vi "CheckForMaxNumberOfOpenFiles.vi"(8 "error in (no error)":errorcluster, 9 "data":T1, 10 "data event":T6, 11 "config":T5) -> (0 "error out":errorcluster, 3 "ok to open new file":bool)   [LabVIEW 2017, in "McsaDataEventCreator.lvlib"]
uses:
  <vilib>/addons/InsightCM/Devices/Shared/Mcsa/McsaDataEventCreator/McsaDataEventCreator.lvlib
  <vilib>/addons/InsightCM/Devices/Shared/Mcsa/McsaDataEventCreator/controls/DataEventConfig.ctl
  <vilib>/addons/InsightCM/Devices/Shared/Mcsa/McsaDataEventCreator/controls/AcqParams.ctl
  <vilib>/addons/InsightCM/Devices/Shared/Common/DataAccumulator/controls/AccumulationSettings.ctl
  <vilib>/addons/InsightCM/Devices/Shared/Common/DataAccumulator/controls/accumulationType.ctl
  <vilib>/addons/InsightCM/Devices/Shared/Common/DVRBuffer/controls/BufferLocation.ctl
  <vilib>/addons/PointValueMap/controls/PointMap.ctl
  <vilib>/addons/InsightCM/Devices/Shared/Mcsa/McsaDataEventCreator/controls/config.ctl
  <vilib>/addons/InsightCM/Devices/Shared/Common/DataFlow/controls/Data.ctl
  <vilib>/addons/InsightCM/Utilities/DataAccessors/controls/wfmSGL_DVR.ctl
  <vilib>/addons/InsightCM/Devices/Shared/Common/DataFlow/controls/Type.ctl
  <vilib>/addons/PointValueMap/PointValueMap.lvlib
  <vilib>/addons/InsightCM/Devices/Shared/Common/DVRBuffer/DVRBuffer.lvlib
  <vilib>/addons/InsightCM/Devices/Shared/Common/DataAccumulator/DataAccumulator.lvlib
  <vilib>/addons/InsightCM/Devices/Shared/Common/DataFlow/DataFlow.lvlib
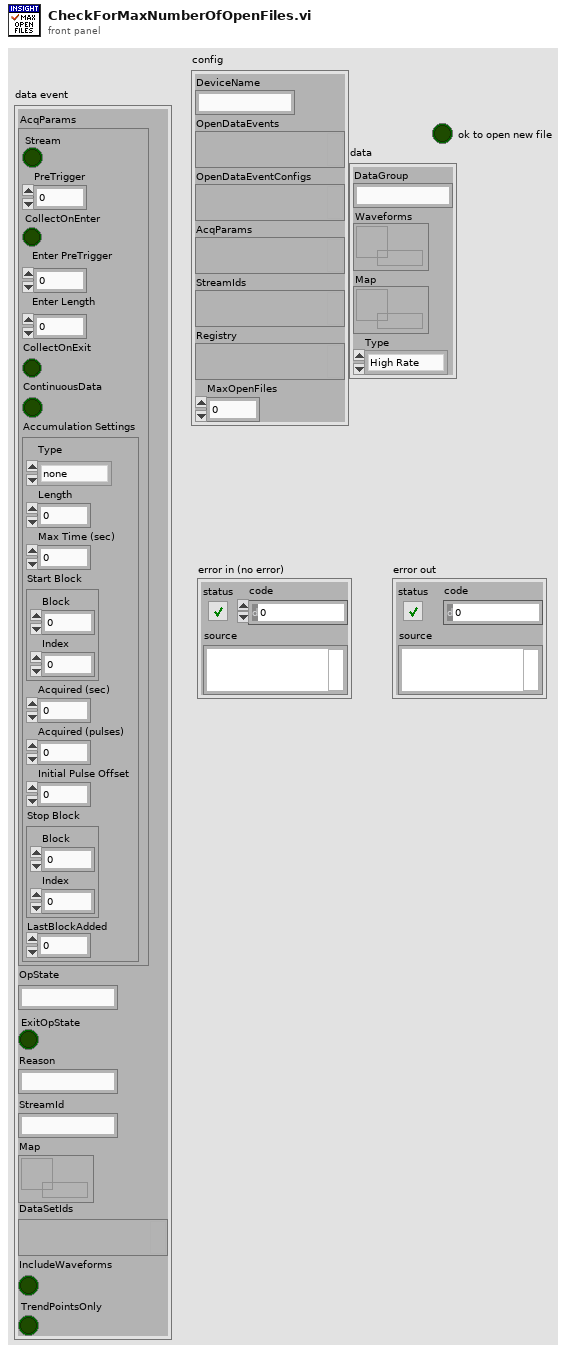
[diagram p1: front panel]
types:
  T1 = typedef "DataFlow.lvlib/Data.ctl" = cluster{"DataGroup":string, "Waveforms":T2, "Map":T3, "Type":T4}
  T2 = typedef "wfmSGL_DVR.ctl" = refnum<data-value>
  T3 = typedef "PointValueMap.lvlib/PointMap.ctl" = refnum<data-value>
  T4 = typedef "DataFlow.lvlib/Type.ctl" = enum16{"High Rate", "Low Rate", "Burst Mode"}
  T5 = typedef "McsaDataEventCreator.lvlib/config.ctl" = cluster{"DeviceName":string, "OpenDataEvents":variant, "OpenDataEventConfigs":variant, "AcqParams":variant, "StreamIds":variant, "Registry":variant, "MaxOpenFiles":i32}
  T6 = typedef "McsaDataEventCreator.lvlib/DataEventConfig.ctl" = cluster{"AcqParams":T7, "OpState":string, "ExitOpState":bool, "Reason":string, "StreamId":string, "Map":T3, "DataSetIds":variant, "IncludeWaveforms":bool, "TrendPointsOnly":bool}
  T7 = typedef "McsaDataEventCreator.lvlib/AcqParams.ctl" = cluster{"Stream":bool, "PreTrigger":i32, "CollectOnEnter":bool, "Enter PreTrigger":i32, "Enter Length":dbl, "CollectOnExit":bool, "ContinuousData":bool, "Accumulation Settings":T8}
  T8 = typedef "DataAccumulator.lvlib/AccumulationSettings.ctl" = cluster{"Type":T9, "Length":dbl, "Max Time (sec)":dbl, "Start Block":T10, "Acquired (sec)":dbl, "Acquired (pulses)":i32, "Initial Pulse Offset":dbl, "Stop Block":T10, "LastBlockAdded":u32}
  T9 = typedef "DataAccumulator.lvlib/accumulationType.ctl" = enum16{"none", "seconds", "revolutions"}
  T10 = typedef "DVRBuffer.lvlib/BufferLocation.ctl" = cluster{"Block":u32, "Index":i32}
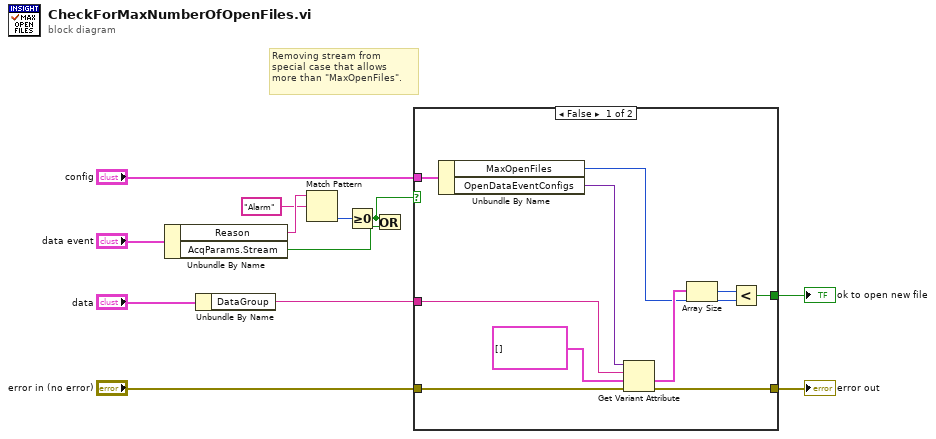
[diagram p0: block diagram]
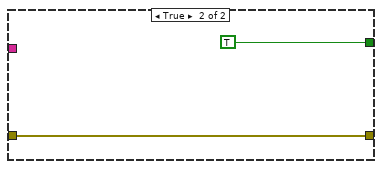
[diagram p2: hidden frame]
diagram:
  # "Removing stream from\nspecial case that allows\nmore than \"MaxOpenFiles\"."
  n1 = Unbundle By Name("data event") -> ("Reason"=w6:string, "AcqParams.Stream"=w7:bool)
  n2 = Unbundle By Name("data") -> ("DataGroup"=w2:string)
  n3 = Match Pattern(string=w6, regular expression="Alarm" ("x")) -> (offset past match=w4:i32)  [unwired: 1 in, 3 out]
  n4 = Greater Or Equal To 0?(x=w4) -> (x >= 0?=w1:bool)
  n5 = Or(x=w1, y=w7) -> ()  [unwired: 1 out]
  n6 = case shown="False" w1 {
    tunnel: [w18 w24] -> w11
    tunnel: "error in (no error)" -> [w21 w24]
    tunnel: [w15 TRUE ("ok to open new file")] -> w9
    tunnel: "config" -> [w20 _]
    tunnel: w2 -> [w14 _]
    frame False {
      n7 = Unbundle By Name(w20) -> ("MaxOpenFiles"=w13:i32, "OpenDataEventConfigs"=w19:variant)
      n8 = Get Variant Attribute(Variant=w19, name=w14, default value (empty Variant)=T6[] [], error in=w21) -> (value=w17:T6[], error out=w18:errorcluster)  [unwired: 2 out]
      n9 = Array Size(array=w17) -> (size(s)=w16:i32)
      n10 = Less?(x=w16, y=w13) -> (x < y?=w15:bool)
    }
    frame True {
    }
  }
  "ok to open new file" <- w9
  "error out" <- w11
